vi "Mapping Data Read.vi"(8 "error constant":errorcluster, 10 "Small File name":string="QS", 11 "Path":path=path "E:/Documents/lab/Maps") -> (0 "error out":errorcluster, 2 "all rows":dbl[][][][](array[numeric]))   [LabVIEW 2012]
doc: "This VI Takes a two letter name (QS) and finds 36 files named E:\\Documents\\lab\\QS\\OQS##LE.DAT\nwhere ## are [A,F][A,F]. It then builds a 4D array:\n1 X position on sample (0-5 for [A,F])\n2 Y position on sample (same as above)\n3 index of array (0- 511 one for each pixel)\n4 Rcm-1 and Counts at that index (0 or 1)"
uses:
  <vilib>/Utility/file.llb/Read From Spreadsheet File (DBL).vi
panel:
  out "XY Graph":cluster{"Y":dbl[], "Y":dbl[]}[](graph)
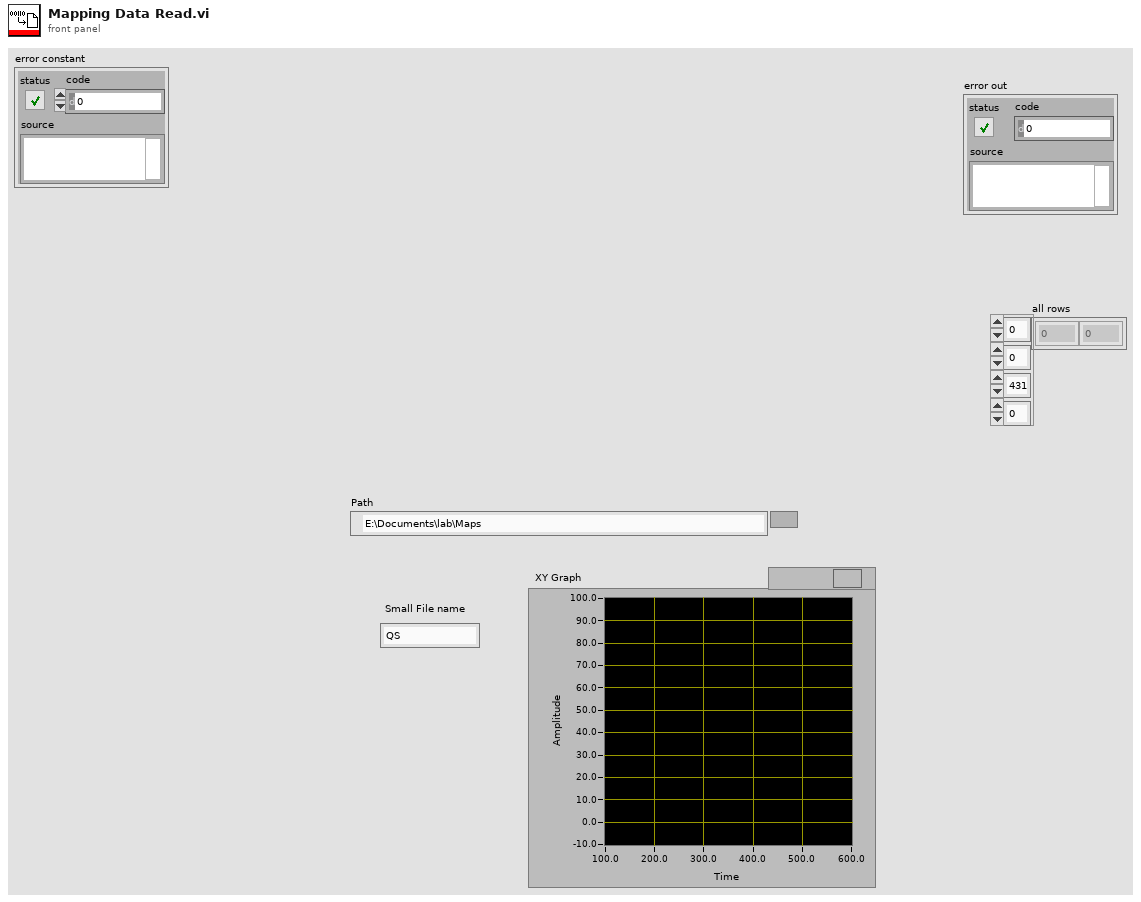
[diagram p1: front panel]
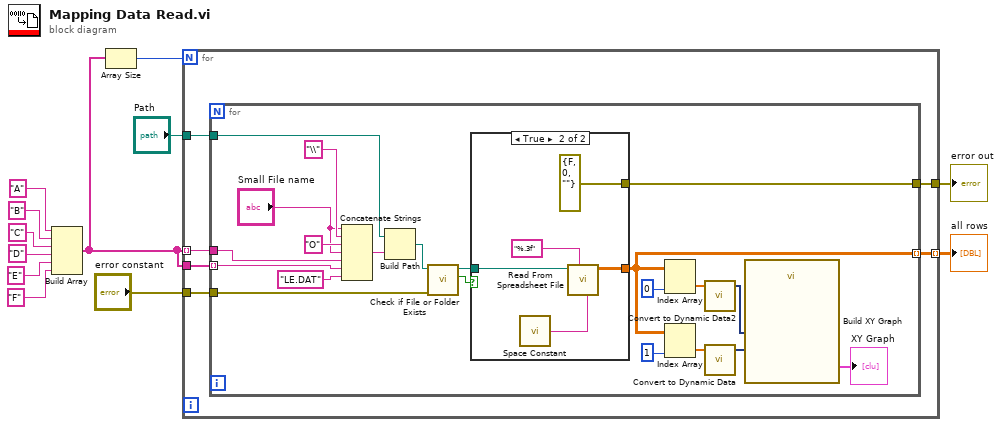
[diagram p0: block diagram]
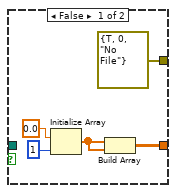
[diagram p2: hidden frame]
diagram:
  n1 = Build Array("A", "B", "C", "D", "E", "F") -> (w5:string[])
  n2 = Array Size(array=w5) -> (size(s)=w12:i32)
  n3 = for {
    N: w12 -> [_]
    tunnel: w5 -> [w18]
    tunnel: w5 -> [w17] mode=indexing
    tunnel: "Path" -> [w16]
    tunnel: [w15] -> w3 mode=indexing
    tunnel: "error constant" -> [w14]
    tunnel: [w13] -> w1
    n4 = for {
      tunnel: w18 -> [w29] mode=indexing
      tunnel: w17 -> [w28]
      tunnel: w16 -> [w25]
      tunnel: [w22] -> w15 mode=indexing
      tunnel: w14 -> [w20]
      tunnel: [w19] -> w13
      n5 = Concatenate Strings("Small File name", "\\", "O", "Small File name", w28, w29, "LE.DAT") -> (w26:string)
      n6 = Build Path(base path=w25, name or relative path=w26) -> (appended path=w24:path)
      n7 = call <vilib>:"Check if File or Folder Exists.vi"("error in (no error)"=w20, "path"=w24) -> ("file or folder exists?"=w23:bool, "dup path"=w21:path)  [unwired: 7 in, 1 out]
      n8 = case shown="True" w23 {
        tunnel: [w41 w47] -> w22
        tunnel: w21 -> [_ w46]
        tunnel: [errorcluster {"status"=TRUE, "code"=0, "source"="No File"} ("error constant") errorcluster {"status"=FALSE, "code"=0, "source"=""} ("error constant")] -> w19
        frame False {
          n9 = Initialize Array(0.0 ("element"), 1 ("dimension size")) -> (w42:dbl[])
          n10 = Build Array(w42, w42) -> (w41:dbl[][])
        }
        frame True {
          n11 = call <vilib>:"Space Constant.vi"() -> ("String"=w48:string)
          n12 = call-poly <vilib>:"Read From Spreadsheet File.vi"("delimiter (\\t)"=w48, "format (%.3f)"="%.3f", "file path (dialog if empty)"=w46) -> ("all rows"=w47:dbl[][])  [unwired: 4 in, 4 out]
        }
      }
      n13 = Index Array(array=w22, index (col)=0 ("index (row)")) -> (element=w36:dbl[])  [unwired: 1 in]
      n14 = Index Array(array=w22, index (col)=1 ("index (row)")) -> (element=w34:dbl[])  [unwired: 1 in]
      n15 = call "Convert to Dynamic Data2"("Array"=w36) -> ("Dynamic Data Type"=w37:dynamicdata)  [unwired: 3 in]
      n16 = call "Convert to Dynamic Data"("Array"=w34) -> ("Dynamic Data Type"=w35:dynamicdata)  [unwired: 3 in]
      n17 = call "Build XY Graph"("Y Input"=w35, "X Input"=w37) -> ("XY Graph"=→"XY Graph":cluster{"Y":dbl[], "Y":dbl[]}[])  [unwired: 3 in, 6 out]
    }
  }
  "all rows" <- w3
  "error out" <- w1
